vi "Force Remove Item.vi"(8 "error in":errorcluster, 11 "item ref":u64) -> (0 "error out":errorcluster)   [LabVIEW 2017, in "Import Export.lvlib"]
uses:
  Import Export.lvlib
  System Explorer Action.ctl
  NationalInstruments.VeriStand.SystemStorage
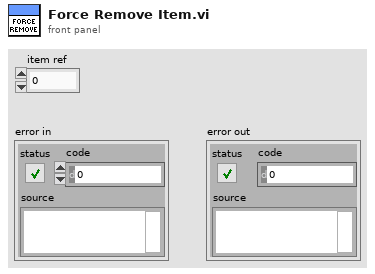
[diagram p1: front panel]
types:
  T1 = typedef "Import Export.lvlib/System Explorer Action.ctl" = u16
  T2 = typedef "Custom Device API.lvlib/Custom Device Item Ref.ctl" = u64
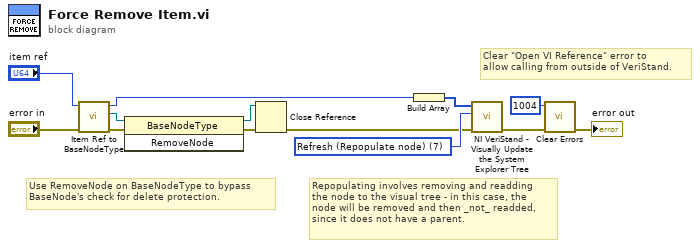
[diagram p0: block diagram]
diagram:
  w10 = T1 7 items=["Refresh (Add)"=5, "Refresh (Repopulate node)"=7, "Refresh (Delete)"=9] ("Action")
  # "Clear \"Open VI Reference\" error to\nallow calling from outside of VeriStand."
  # "Use RemoveNode on BaseNodeType to bypass\nBaseNode's check for delete protection."
  # "Repopulating involves removing and readding\nthe node to the visual tree - in this case, the\nnode will be removed and then _not_ readded,\nsince it does not have a parent."
  n1 = call "Item Ref to BaseNodeType.vi"("error in (no error)"="error in", "item ref in"="item ref") -> ("error out"=w1:errorcluster, "BaseNodeType"=w2:refnum<k24>, "item ref out"=w3:T2)  [unwired: 7 in]
  n2 = invoke class="BaseNodeType" method="RemoveNode"(reference=w2, error in=w1) -> (reference out=w12:refnum<k24>, error out=w13:errorcluster)  [unwired: 1 in, 1 out]
  n3 = Close Reference(reference=w12, error in (no error)=w13) -> (error out=w8:errorcluster)
  n4 = Build Array(w3) -> (w11:T2[])
  n5 = call "NI VeriStand - Visually Update the System Explorer Tree.vi"("error in (no error)"=w8, "Action"=w10, "Node IDs"=w11) -> ("error out"=w7:errorcluster)  [unwired: 8 in]
  n6 = call <vilib>:"Clear Errors.vi"("error in (no error)"=w7, "specific error code to clear (0: all)"=1004) -> ("error out"=→"error out":errorcluster)  [unwired: 4 in, 1 out]
